vi "RSZVB Channel Rename.vi"(8 "error in (no error)":errorcluster {"code" format="%.0x"}, 9 "Channel Name (Chan1)":string="Chan1", 10 "Channel (1)":i32=1, 11 "VISA session":refnum<visa-resource-name>) -> (0 "error out":errorcluster {"code" format="%.0x"}, 3 "dup VISA session":refnum<visa-resource-name>)   [LabVIEW 2011]
doc: "This VI assigns a name to channel number. The channel must be created before. Moreover it is not possible to assign the same name to two different channels.\n\nRemote-control command(s):\nCONFigure:CHANnel<Ch>:NAME '<Ch_name>'"
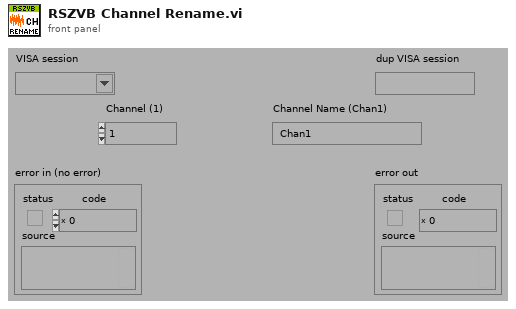
[diagram p1: front panel]
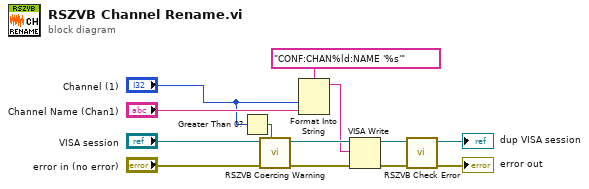
[diagram p0: block diagram]
diagram:
  n1 = Greater Than 0?(x="Channel (1)") -> (x > 0?=w9:bool)
  n2 = call "RSZVB Coercing Warning.vi"("In Range?"=w9, "error in (no error)"="error in (no error)", "VISA session"="VISA session") -> ("error out"=w12:errorcluster, "dup VISA session"=w13:refnum<visa-resource-name>)  [unwired: 7 in]
  n3 = Format Into String(format string="CONF:CHAN%ld:NAME '%s'", "Channel (1)", "Channel Name (Chan1)") -> (resulting string=w1:string)  [unwired: 2 in, 1 out]
  n4 = VISA Write(VISA resource name=w13, write buffer=w1, error in (no error)=w12) -> (VISA resource name out=w10:refnum<visa-resource-name>, error out=w11:errorcluster)  [unwired: 1 out]
  n5 = call "RSZVB Check Error.vi"("error in (no error)"=w11, "VISA session"=w10) -> ("error out"=→"error out":errorcluster, "dup VISA session"=→"dup VISA session":refnum<visa-resource-name>)  [unwired: 8 in]
